vi "MotorenAnsteuern_Dateneinlesen.vi"() -> ()   [LabVIEW 2023]
panel:
  in  "Handshake 2":bool
  in  "Standby":bool
  in  "Inhibit":bool
  in  "Reserviert 7":bool
  in  "Reservier":bool
  in  "AS2 aktivieren":bool
  in  "Reserviert 2":bool
  in  "Fehler_Reset":bool
  in  "Start":bool
  in  "Reserviert 3":bool
  in  "Reserviert 4":bool
  in  "Reserviert 5":bool
  in  "Bremse öffnen":bool
  in  "Reserviert 6":bool
  in  "Enable/ApplicationStop":bool
  in  "Enable/EmergencyStop":bool
  out "Numeric":i32
  in  "Speed":dbl
  out "size(s)":i32[](array[numeric])
  in  "file (use dialog)":path
  out "IP Adresse":string
  in  "Motor auswählen":string(combo)
  out "Digital":dbl
  out "Drehmoment":dbl
  out "Status/Fehler":dbl
  out "Istgeschwindigkeit":dbl
  out "Handshake":bool
  out "Standby aktiv":bool
  out "Reserviert":bool
  out "SWES inaktiv":bool
  out "Geschwindigkeit erreicht":bool
  out "AS2 aktiv":bool
  out "Warnung":bool
  out "Fehler":bool
  out "in Position":bool
  out "Relativposition übernommen":bool
  out "referenziert":bool
  out "Motor dreht":bool
  out "Bremse geöffnet":bool
  out "Endstufenfreigabe":bool
  out "STO inaktiv":bool
  out "Betriebsbereit":bool
  in  "Stopp":bool
  in  "Digital":dbl
  in  "Deceleration":dbl
  in  "Acceleration":dbl
  # "zum MOVIDRIVE"
  # "vom MOVIDRIVE"
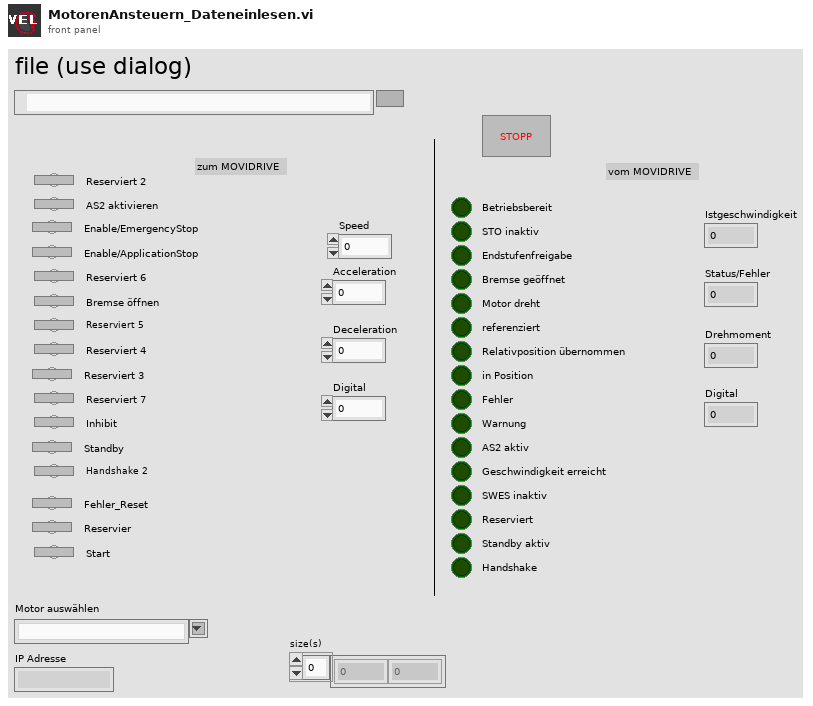
[diagram p1: front panel]
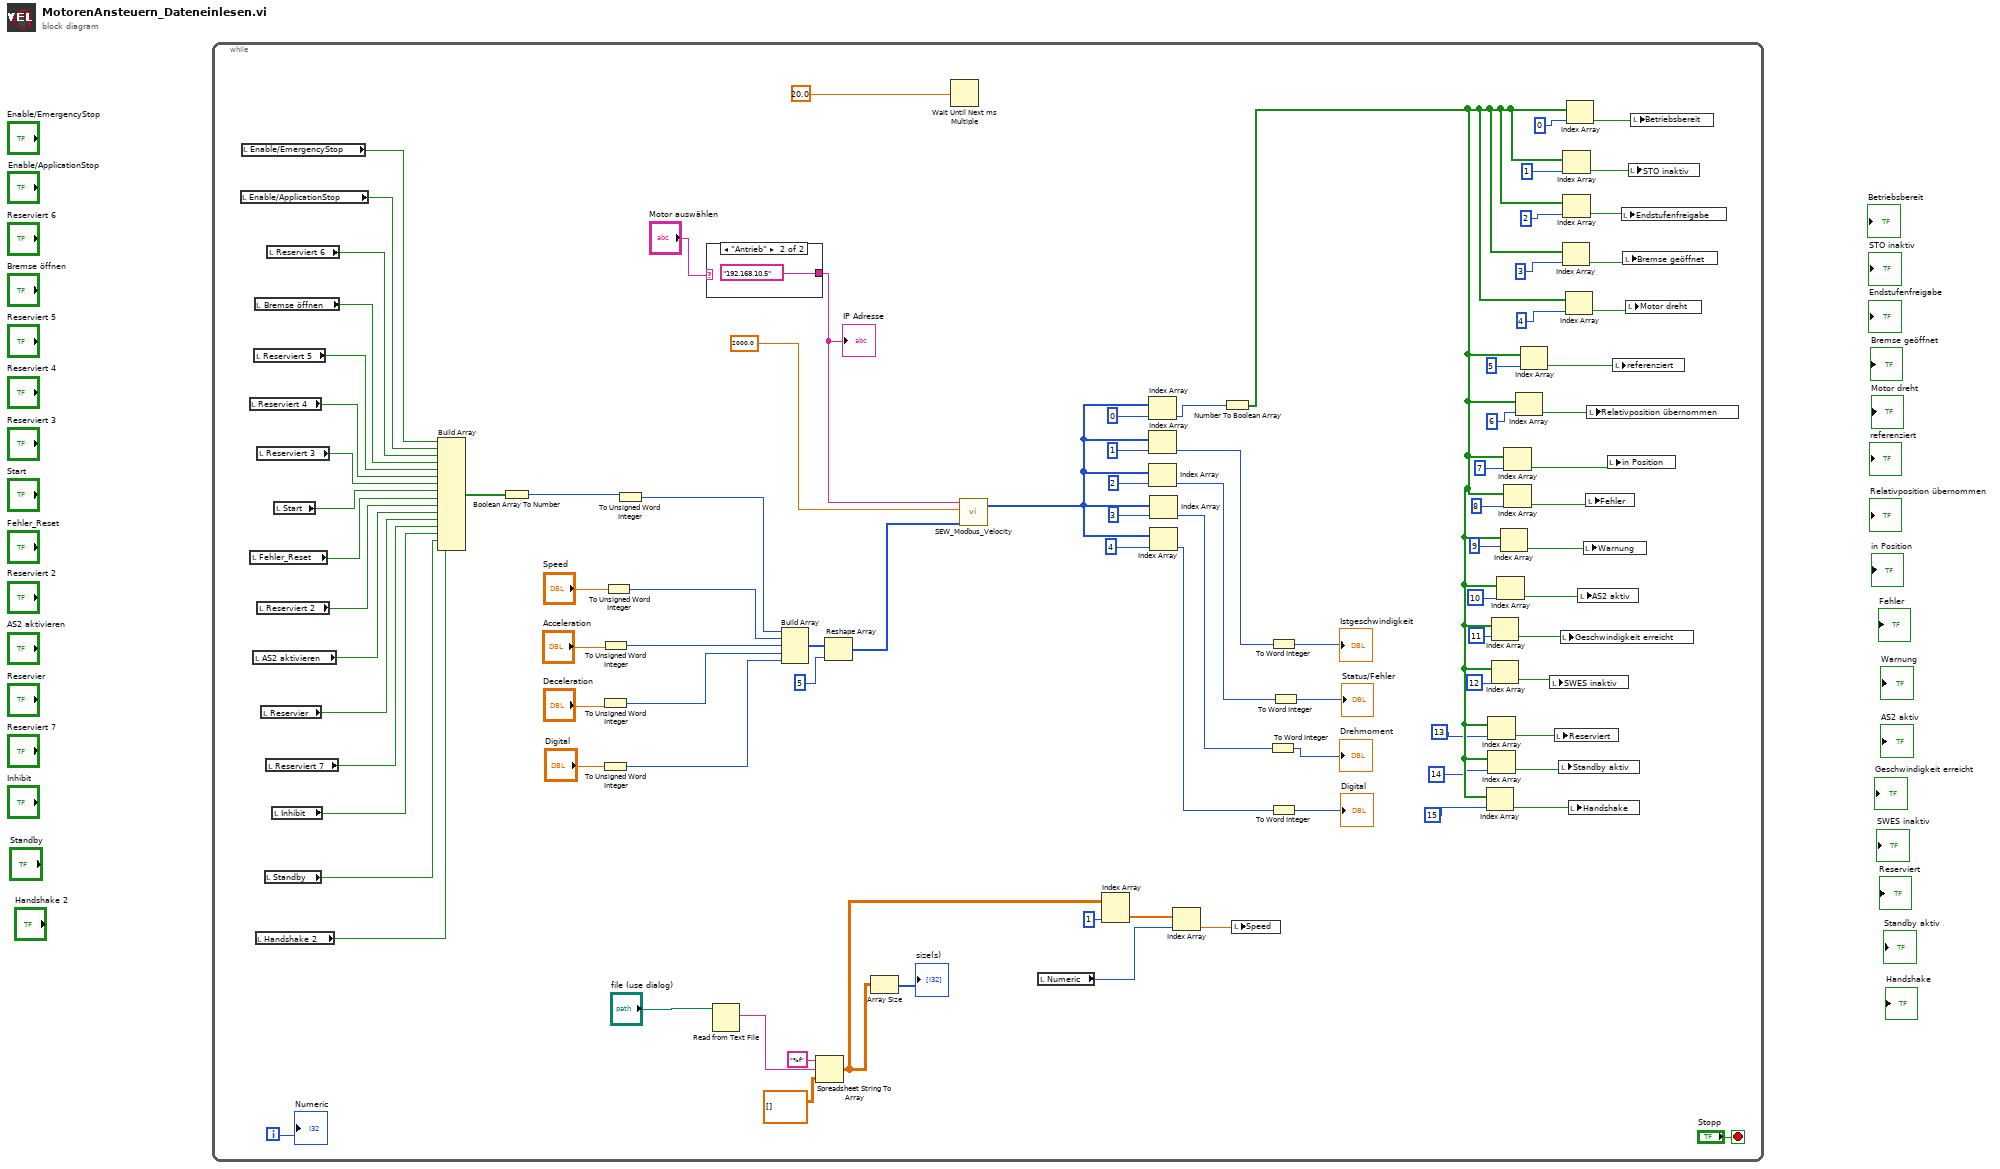
[diagram p0: block diagram]
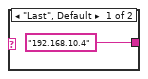
[diagram p2: hidden frame]
diagram:
  n1 = while {
    i -> [w43]
    stop <- "Stopp" stop-if-true
    n2 = local read "Enable/ApplicationStop"() -> (w15:bool)
    n3 = local read "Enable/EmergencyStop"() -> (w16:bool)
    n4 = local read "Reserviert 4"() -> (w11:bool)
    n5 = local read "Fehler_Reset"() -> (w2:bool)
    n6 = local read "AS2 aktivieren"() -> (w4:bool)
    n7 = local read "Reserviert 5"() -> (w12:bool)
    n8 = local read "Bremse öffnen"() -> (w13:bool)
    n9 = local read "Handshake 2"() -> (w9:bool)
    n10 = local read "Reserviert 3"() -> (w10:bool)
    n11 = local read "Reserviert 2"() -> (w3:bool)
    n12 = local read "Reservier"() -> (w5:bool)
    n13 = local read "Standby"() -> (w8:bool)
    n14 = local read "Reserviert 7"() -> (w6:bool)
    n15 = local read "Reserviert 6"() -> (w14:bool)
    n16 = local read "Inhibit"() -> (w7:bool)
    n17 = local read "Start"() -> (w1:bool)
    n18 = Build Array(w16, w15, w14, w13, w12, w11, w10, w1, w2, w3, w4, w5, w6, w7, w8, w9) -> (w83:bool[])
    n19 = Boolean Array To Number(Boolean array=w83) -> (number=w84:u32)
    n20 = To Unsigned Word Integer(number="Deceleration") -> (unsigned 16bit integer=w90:u16)
    n21 = To Unsigned Word Integer(number="Digital") -> (unsigned 16bit integer=w91:u16)
    n22 = To Unsigned Word Integer(number="Acceleration") -> (unsigned 16bit integer=w89:u16)
    n23 = To Unsigned Word Integer(number="Speed") -> (unsigned 16bit integer=w92:u16)
    n24 = To Unsigned Word Integer(number=w84) -> (unsigned 16bit integer=w88:u16)
    n25 = case shown="\"Antrieb\"" "Motor auswählen" {
      tunnel: ["192.168.10.4" "192.168.10.5"] -> w45
      frame "Last", Default {
      }
      frame "Antrieb" {
      }
    }
    "IP Adresse" <- w45
    n26 = Read from Text File(file (use dialog)="file (use dialog)") -> (text=w38:string)  [unwired: 2 in, 4 out]
    n27 = Build Array(w88, w92, w89, w90, w91) -> (w93:u16[])
    n28 = Spreadsheet String To Array(format string="%f", spreadsheet string=w38, array type (2D Dbl)=dbl[][] []) -> (array=w33:dbl[][])  [unwired: 1 in]
    n29 = Reshape Array(w93, 5) -> (w80:u16[])
    n30 = Array Size(array=w33) -> (size(s)=→"size(s)":i32[])
    n31 = Wait Until Next ms Multiple(millisecond multiple=20.0 ("Update(ms)")) -> ()  [unwired: 1 out]
    n32 = call "SEW_Modbus_Velocity.vi"("Remote IP Address"=w45, "Timeout [ms]"=2000.0 ("Timeout (ms)"), "Output (Write Multiple Register) 2"=w80) -> ("Input (Read Holding Register) 2"=w78:u16[])  [unwired: 3 in]
    n33 = local read "Numeric"() -> (w42:i32)
    n34 = Index Array(array=w33, index (col)=1 ("disabled index (col)")) -> (element=w41:dbl[])  [unwired: 1 in]
    n35 = Index Array(array=w78, index=0) -> (element=w64:u16)
    n36 = Index Array(array=w78, index=1) -> (element=w65:u16)
    n37 = Index Array(array=w78, index=2) -> (element=w66:u16)
    n38 = Index Array(array=w78, index=3) -> (element=w67:u16)
    n39 = Index Array(array=w78, index=4) -> (element=w68:u16)
    n40 = Index Array(array=w41, index=w42) -> (element=w40:dbl)
    n41 = Number To Boolean Array(number=w64) -> (Boolean array=w63:bool[])
    n42 = local write "Speed"(w40) -> ()
    n43 = To Word Integer(number=w67) -> (16bit integer=→"Drehmoment":i16)
    n44 = To Word Integer(number=w65) -> (16bit integer=→"Istgeschwindigkeit":i16)
    n45 = To Word Integer(number=w68) -> (16bit integer=→"Digital":i16)
    n46 = To Word Integer(number=w66) -> (16bit integer=→"Status/Fehler":i16)
    n47 = Index Array(array=w63, index=15) -> (element=w17:bool)
    n48 = Index Array(array=w63, index=13) -> (element=w19:bool)
    n49 = Index Array(array=w63, index=14) -> (element=w18:bool)
    n50 = Index Array(array=w63, index=11) -> (element=w21:bool)
    n51 = Index Array(array=w63, index=12) -> (element=w20:bool)
    n52 = Index Array(array=w63, index=10) -> (element=w22:bool)
    n53 = Index Array(array=w63, index=9) -> (element=w23:bool)
    n54 = Index Array(array=w63, index=7) -> (element=w25:bool)
    n55 = Index Array(array=w63, index=8) -> (element=w24:bool)
    n56 = Index Array(array=w63, index=6) -> (element=w26:bool)
    n57 = Index Array(array=w63, index=5) -> (element=w27:bool)
    n58 = local write "SWES inaktiv"(w20) -> ()
    n59 = local write "Reserviert"(w19) -> ()
    n60 = local write "Standby aktiv"(w18) -> ()
    n61 = local write "Geschwindigkeit erreicht"(w21) -> ()
    n62 = Index Array(array=w63, index=3) -> (element=w29:bool)
    n63 = Index Array(array=w63, index=1) -> (element=w31:bool)
    n64 = Index Array(array=w63, index=2) -> (element=w30:bool)
    n65 = Index Array(array=w63, index=4) -> (element=w28:bool)
    n66 = Index Array(array=w63, index=0) -> (element=w32:bool)
    n67 = local write "Handshake"(w17) -> ()
    n68 = local write "AS2 aktiv"(w22) -> ()
    n69 = local write "Warnung"(w23) -> ()
    n70 = local write "Fehler"(w24) -> ()
    n71 = local write "Relativposition übernommen"(w26) -> ()
    n72 = local write "in Position"(w25) -> ()
    n73 = local write "referenziert"(w27) -> ()
    n74 = local write "Endstufenfreigabe"(w30) -> ()
    n75 = local write "Bremse geöffnet"(w29) -> ()
    n76 = local write "Motor dreht"(w28) -> ()
    n77 = local write "STO inaktiv"(w31) -> ()
    n78 = local write "Betriebsbereit"(w32) -> ()
    "Numeric" <- w43
  }
